vi "Reading From Modbus Registers.vi"(8 "error in (no error)":errorcluster caption="错误输入（无错误）", 11 "Regs Address":u16[](array[numeric])) -> (0 "error out":errorcluster caption="错误输出", 3 "Input Registers":u16[](array[numeric]))   [LabVIEW 2010]
uses:
  Source Code/SubVIs/NI Modbus.llb/MB Serial Master Query Read Input Registers (poly).vi
  SubVIs/Controller Communication.llb/F4 Controller handle Global Function Enum.ctl
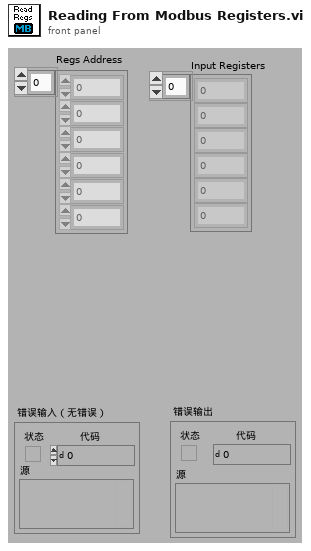
[diagram p1: front panel]
types:
  T1 = cluster{"Mode":enum16{"RTU", "ASCII"}, "Slave Address":u8}
  T2 = typedef "F4 Controller handle Global Function Enum.ctl" = enum16{"保存信息", "读取信息", "读取控制器列表", "选择控制器", "初始化"}
  T3 = typedef "F4 Controller handle.ctl" = cluster{"F4Ctrller Name":string, "Ctrller Address":i32, "VISA handle":refnum<visa-resource-name>}
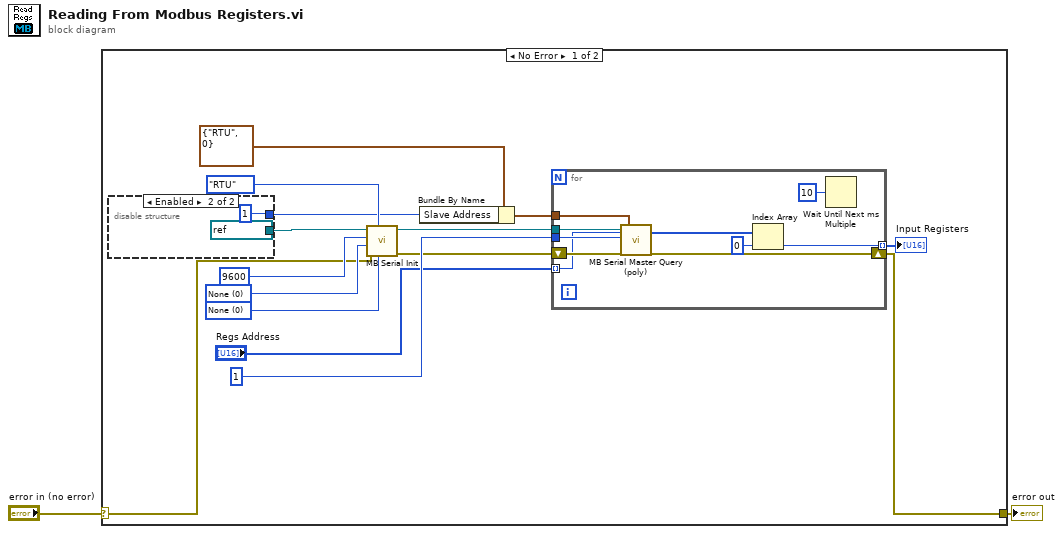
[diagram p0: block diagram]
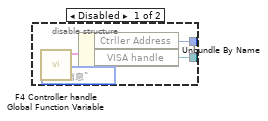
[diagram p2: hidden frame]
diagram:
  n1 = case shown="No Error" "error in (no error)" {
    selector: "error in (no error)" -> [w6 w34]
    tunnel: [w5 w34] -> w1
    frame No Error {
      w15 = u16 0 items=["None", "XON/XOFF", "RTS/CTS", "XON/XOFF & RTS/CTS", "DTR/DSR", "XON/XOFF & DTR/DSR"] ("Flow Control")
      w14 = u16 0 items=["None", "Odd", "Even", "Mark", "Space"] ("Parity")
      n2 = disable-structure shown="Enabled" {
        disable-tunnel: [w21 refnum<visa-resource-name> "COM1" ("VISA resource name")] -> w11
        disable-tunnel: [w20 1 ("Ctrller Address")] -> w10
        frame Disabled {
          n3 = call "F4 Controller handle Global Function Variable.vi"("F4 Controller handle Global Function Enum"=F4_Controller_handle_Global_Function_Enum."读取信息") -> ("控制器信息"=w19:T3)  [unwired: 7 in, 3 out]
          n4 = Unbundle By Name(w19) -> ("Ctrller Address"=w20:i32, "VISA handle"=w21:refnum<visa-resource-name>)
        }
        frame Enabled {
        }
      }
      n5 = call "MB Serial Init.vi"("Flow Control"=w15, "Mode"=enum16{"RTU", "ASCII"}."RTU", "error in (no error)"=w6, "Parity"=w14, "Baud Rate"=u32 9600, "VISA resource name"=w11) -> ("error out"=w16:errorcluster, "VISA resource name out"=w7:refnum<visa-resource-name>)  [unwired: 4 in]
      n6 = Bundle By Name(cluster=T1 {"Mode"=enum."RTU", "Slave Address"=0} ("Serial Parameters"), "Slave Address"=w10) -> (w9:T1)
      n7 = for {
        tunnel: u16 1 ("Quantity") -> [w31]
        tunnel: w9 -> [w29]
        tunnel: w7 -> [w28]
        tunnel: "Regs Address" -> [w26] mode=indexing
        tunnel: [w24] -> w3 mode=indexing
        shift-right: [w27] -> w5
        shift-left: w16 -> [w30]
        n8 = call-poly "MB Serial Master Query (poly).vi"("VISA resource name"=w28, "Starting Address"=w26, "Quantity"=w31, "error in"=w30, "Serial Parameters"=w29) -> ("Input Registers"=w32:u16[], "error out"=w27:errorcluster)  [unwired: 11 in, 2 out]
        n9 = Index Array(array=w32, index=0 ("索引")) -> (element=w24:u16)
        n10 = Wait Until Next ms Multiple(millisecond multiple=u32 10 ("毫秒倍数")) -> ()  [unwired: 1 out]
      }
      "Input Registers" <- w3
    }
    frame Error {
    }
  }
  "error out" <- w1
